vi "SettingButton_MenuSelect.vi"(8 "error in (no error)":errorcluster caption="错误输入（无错误）", 9 "QName":string, 10 "MenuTag":string, 11 "PCM PanelSplit 输入":refnum<class "PCM PanelSplit.lvclass"> caption="DNL_LabVIEW Object in") -> (0 "error out":errorcluster caption="错误输出", 3 "PCM PanelSplit 输出":refnum<class "PCM PanelSplit.lvclass"> caption="DNL_LabVIEW Object out")   [LabVIEW 2016, in "PCM PanelSplit.lvclass"]
uses:
  PCM PanelSplit.lvclass
  Display Mode.ctl
  PanelSplitToolkit/QueueManager.llb/Insert.vi
  GlobleVariables/Ctrl_Sample Configure.ctl
panel:
  out "Channel Changed":bool
  out "DisplayMode Changed":bool
  in  "Display Mode":T1
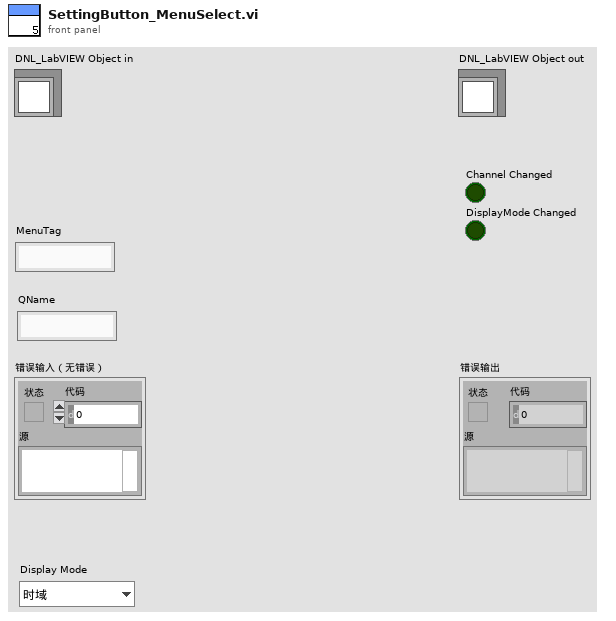
[diagram p1: front panel]
types:
  T1 = typedef "PCM PanelSplit.lvclass/Display Mode.ctl" = enum16{"时域", "频谱", "功率谱"}
  T2 = typedef "Ctrl_Sample Configure.ctl" = enum16{"Read", "Set"}
  T3 = cluster{"SignalType":string[], "Channels Tag":string[], "Channels Name":string[], "Unit":string[], "Alarm Upper Limit":dbl[], "Alarm Lower Limit":dbl[], "Sensitivity":dbl[], "SampleRate":dbl[], "Sensor":string[]}
  T4 = typedef "PCM PanelSplit.lvclass/Display Config.ctl" = cluster{"Display Mode":T1, "ChTag[]":string[], "window":T5, "Range":T6}
  T5 = typedef "NI_AALPro.lvlib/windowTd.ctl" = u32
  T6 = typedef "LVRangeTypeDef.ctl" = cluster{"Minimum":dbl, "Maximum":dbl, "Increment":dbl, "Minor Increment":dbl, "Start":dbl}
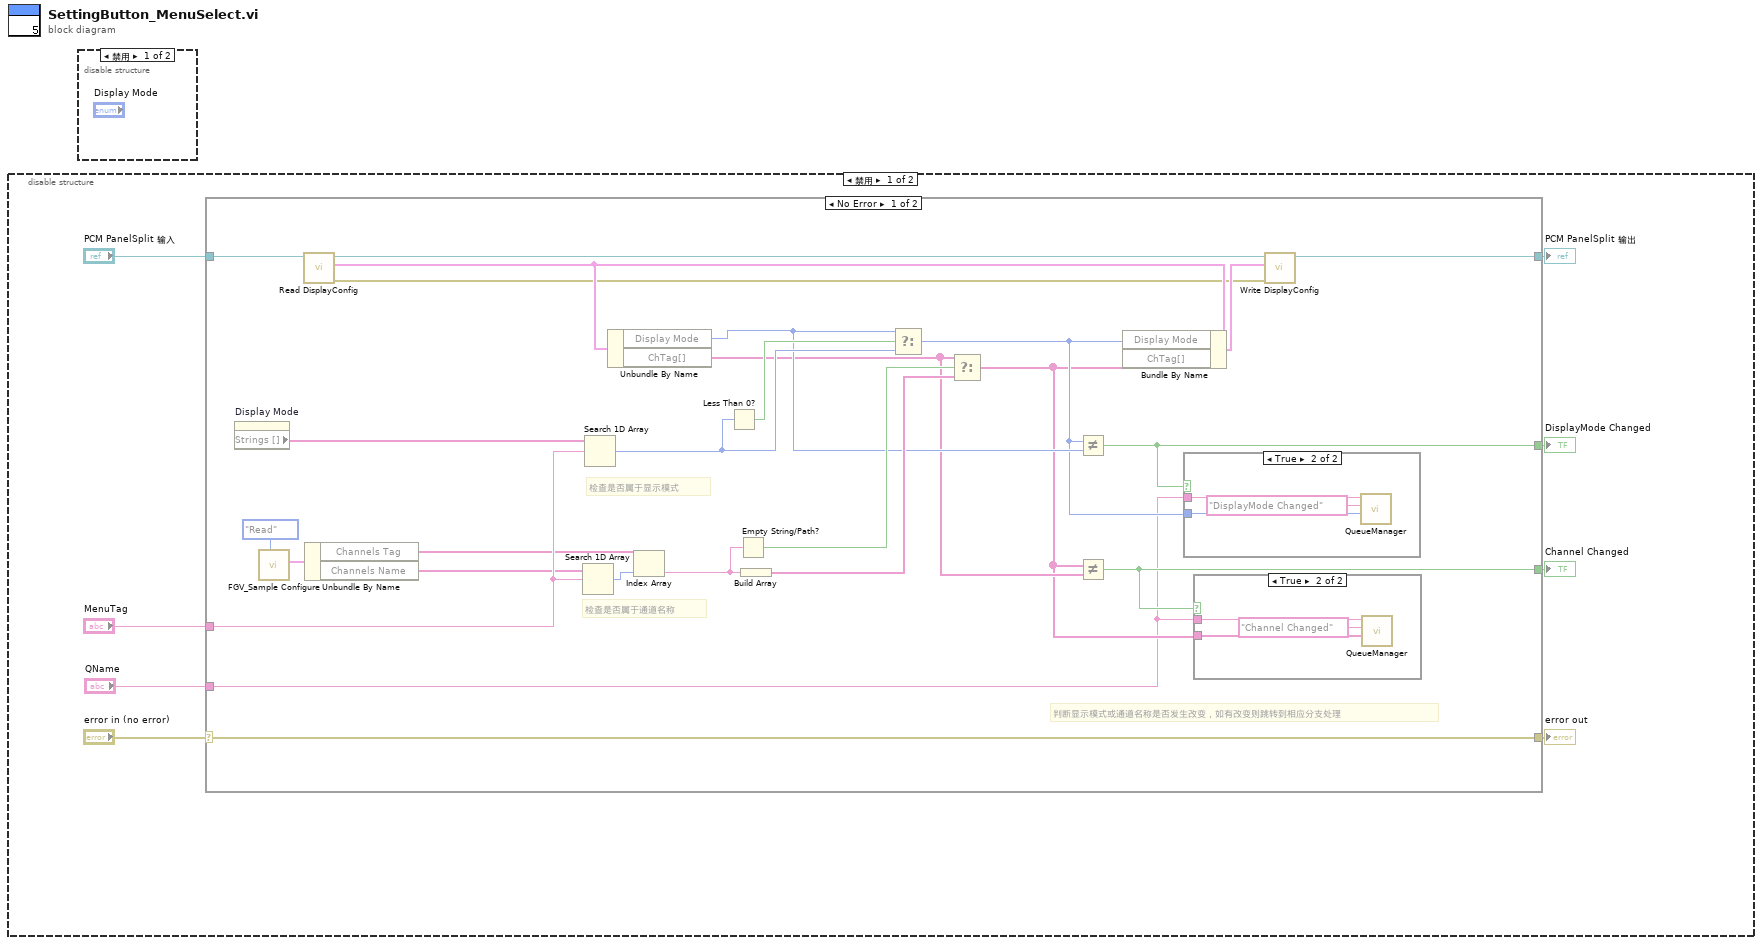
[diagram p0: block diagram]
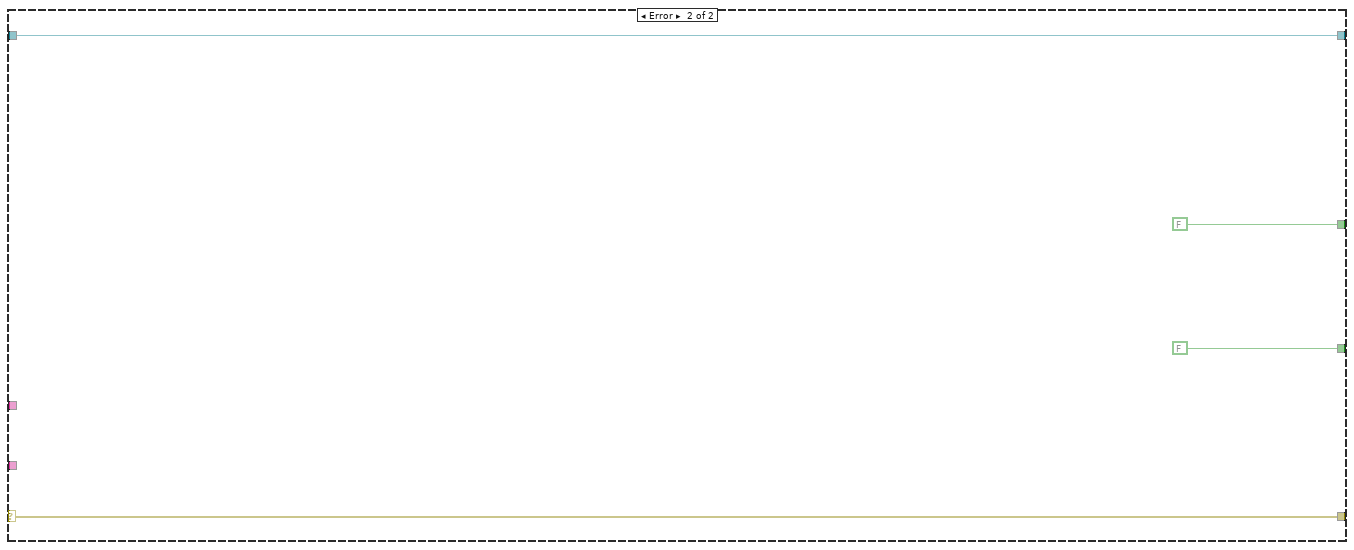
[diagram p4: hidden frame]
diagram:
  n1 = disable-structure shown="禁用" {
    frame Disabled {
      n2 = case shown="No Error" "error in (no error)" {
        selector: "error in (no error)" -> [w34 w44]
        tunnel: [w34 w44] -> w7
        tunnel: [w31 w43] -> w5
        tunnel: "PCM PanelSplit 输入" -> [w33 w43]
        tunnel: "MenuTag" -> [w18 _]
        tunnel: [w17 FALSE] -> w3
        tunnel: [w14 FALSE] -> w2
        tunnel: "QName" -> [w13 _]
        frame No Error {
          # "判断显示模式或通道名称是否发生改变，如有改变则跳转到相应分支处理"
          # "检查是否属于通道名称"
          # "检查是否属于显示模式"
          n3 = property on="Display Mode" class="Enum (strict)"() -> ("Strings []"=w30:string[])  [unwired: 2 in, 2 out]
          n4 = call "FGV_Sample Configure.vi"("Action"=Ctrl_Sample_Configure."Read") -> ("SignalTable"=w12:T3)  [unwired: 9 in, 1 out]
          n5 = call "Read DisplayConfig.vi"("PCM PanelSplit 输入"=w33) -> ("error out"=w21:errorcluster, "Display Config"=w27:T4, "PCM PanelSplit 输出"=w32:refnum<class "PCM PanelSplit.lvclass">)  [unwired: 8 in]
          n6 = Unbundle By Name(w12) -> ("Channels Tag"=w10:string[], "Channels Name"=w9:string[])
          n7 = Search 1D Array(1D array=w9, element=w18) -> (index of element=w28:i32)  [unwired: 1 in]
          n8 = Search 1D Array(1D array=w30, element=w18) -> (index of element=w25:i32)  [unwired: 1 in]
          n9 = Unbundle By Name(w27) -> ("Display Mode"=w20:T1, "ChTag[]"=w19:string[])
          n10 = Index Array(array=w10, index=w28) -> (element=w23:string)
          n11 = Less Than 0?(x=w25) -> (x < 0?=w26:bool)
          n12 = Empty String/Path?(string/path=w23) -> (empty?=w24:bool)
          n13 = Build Array(w23) -> (w22:string[])
          n14 = Select(t=w20, s=w26, f=w25) -> (s? t:f=w16:i32)
          n15 = Select(t=w19, s=w24, f=w22) -> (s? t:f=w15:string[])
          n16 = Not Equal?(x=w16, y=w20) -> (x != y?=w17:bool)
          n17 = Not Equal?(x=w15, y=w19) -> (x != y?=w14:bool)
          n18 = Bundle By Name(cluster=w27, "Display Mode"=w16, "ChTag[]"=w15) -> (w29:T4)
          n19 = case shown="True" w17 {
            tunnel: w16 -> [_ w40]
            tunnel: w13 -> [_ w39]
            frame False {
            }
            frame True {
              n20 = call-poly "QueueManager.vi"("Data"=w40, "Event"="DisplayMode Changed", "QueueName"=w39) -> ()  [unwired: 7 in, 2 out]
            }
          }
          n21 = case shown="True" w14 {
            tunnel: w15 -> [_ w37]
            tunnel: w13 -> [_ w36]
            frame False {
            }
            frame True {
              n22 = call-poly "QueueManager.vi"("Data"=w37, "Event"="Channel Changed", "QueueName"=w36) -> ()  [unwired: 7 in, 2 out]
            }
          }
          n23 = call "Write DisplayConfig.vi"("error in"=w21, "Display Config"=w29, "PCM PanelSplit 输入"=w32) -> ("PCM PanelSplit 输出"=w31:refnum<class "PCM PanelSplit.lvclass">)  [unwired: 7 in, 1 out]
        }
        frame Error {
        }
      }
      "error out" <- w7
      "PCM PanelSplit 输出" <- w5
      "DisplayMode Changed" <- w3
      "Channel Changed" <- w2
    }
    frame Enabled {
    }
  }
  n24 = disable-structure shown="禁用" {
    frame Disabled {
    }
    frame Enabled {
    }
  }
